vi "PH_HamamatsuCamera.set ROI Max Knob.vi"(0 "VI in":refnum<vi>, 5 "error in (no error)":errorcluster) -> (14 "VI out":refnum<vi>, 19 "error out":errorcluster)   [LabVIEW 2014, in "PH_HamamatsuCamera.lvlib"]
doc: "This VI sets several things related to ROI stuff."
uses:
  PH_HamamatsuCamera.lvlib
  PH_Common/PH_Common.lvlib
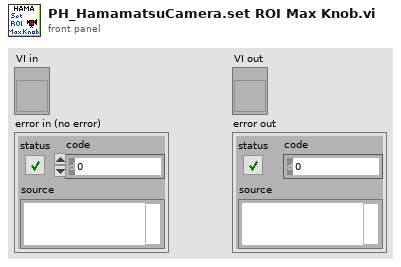
[diagram p1: front panel]
types:
  T1 = typedef "PH_HamamatsuCamera.lvlib/PH_HamamatsuCamera.i attribute.ctl" = cluster{"Gui Refs":cluster{"Camera Details":refnum<vi>, "ROI":refnum<vi>, "Set ROI to Maximum":refnum<vi>, "Trigger Parameters":refnum<vi>, "Brightness":refnum<vi>, "Shutter":refnum<vi>, "Gain":refnum<vi>, "Trigger Timeout":refnum<vi>, "Trigger Polarity":refnum<vi>, "Trigger Mode":refnum<vi>, "Parameters":refnum<vi>, "Set Cam Parameter":refnum<vi>, "Parameter to set":refnum<vi>, "Value to set":refnum<vi>}, "Cam":cluster{"Handle":i32, "Details":cluster{"Model":string, "Camera ID":string, "Firmware":string}, "Buffer Info":cluster{"height":u32, "width":u32, "datatype":u32}}, "H Offset":cluster{"Value":i32, "Minimum":i32, "Maximum":i32, "Increment":i32}, "V Offset":cluster{"Value":i32, "Minimum":i32, "Maximum":i32, "Increment":i32}, "H Width":cluster{"Value":i32, "Minimum":i32, "Maximum":i32, "Increment":i32}, "V Width":cluster{"Value":i32, "Minimum":i32, "Maximum":i32, "Increment":i32}, "Trigger Parameters":T2, "Trigger Timeout":u32, "Parameters":T3[], "Indicees Cam Parameters":cluster{"Brightness":i32, "Shutter":i32, "Gain":i32}, "Wanted Values":cluster{"Trigger Settings":T2[], "ROI":T4[], "Parameter":cluster{"Name":string, "Value":dbl}[]}}
  T2 = typedef "PH_HamamatsuCamera.lvlib/PH_HamamatsuCamera.Trigger Parameter.ctl" = cluster{"Mode":u32, "Polarity":u32, "Times":u32, "Delay":dbl}
  T3 = typedef "PH_HamamatsuCamera.lvlib/PH_HamamatsuCamera.Parameter Set.ctl" = cluster{"Parameter":string, "Value":dbl, "Writable":bool, "Range":cluster{"min":dbl, "max":dbl, "step":dbl}, "Default":dbl, "Value Names":cluster{"Name":string, "Value":dbl}[], "Text Values":bool}
  T4 = typedef "PH_HamamatsuCamera.lvlib/PH_HamamatsuCamera.ROI.ctl" = cluster{"Horizontal Offset":i32, "Vertical Offset":i32, "Horizontal Width":i32, "Vertical Width":i32}
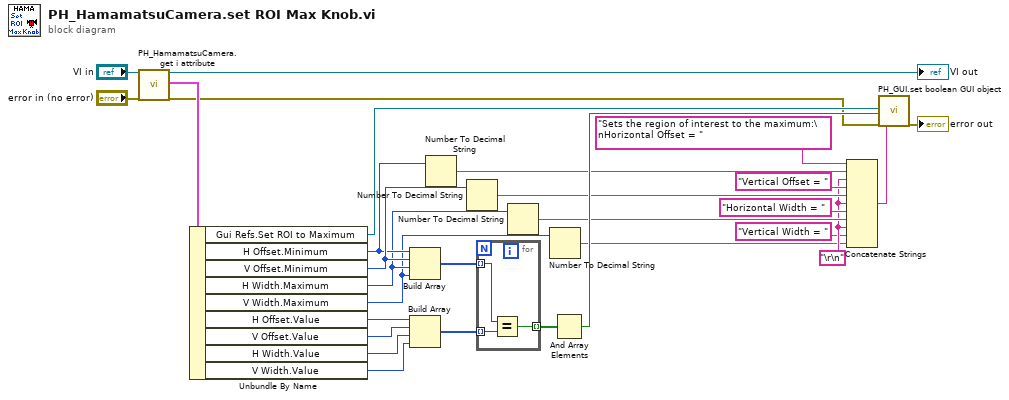
[diagram p0: block diagram]
diagram:
  w11 = "\r\n"
  n1 = call "PH_HamamatsuCamera.get i attribute.vi"("i ref in"="VI in", "error in (no error)"="error in (no error)") -> ("i ref out"=→"VI out":refnum<vi>, "i attribute"=w22:T1, "error out"=w5:errorcluster)  [unwired: 15 in]
  n2 = Unbundle By Name(w22) -> ("Gui Refs.Set ROI to Maximum"=w16:refnum<vi>, "H Offset.Minimum"=w3:i32, "V Offset.Minimum"=w4:i32, "H Width.Maximum"=w2:i32, "V Width.Maximum"=w1:i32, "H Offset.Value"=w23:i32, "V Offset.Value"=w24:i32, "H Width.Value"=w25:i32, "V Width.Value"=w26:i32)
  n3 = Build Array(w3, w4, w2, w1) -> (w17:i32[])
  n4 = Build Array(w23, w24, w25, w26) -> (w27:i32[])
  n5 = Number To Decimal String(number=w3) -> (decimal integer string=w18:string)  [unwired: 1 in]
  n6 = Number To Decimal String(number=w4) -> (decimal integer string=w14:string)  [unwired: 1 in]
  n7 = for {
    tunnel: w27 -> [w32] mode=indexing
    tunnel: w17 -> [w30] mode=indexing
    tunnel: [w31] -> w8 mode=indexing
    n8 = Equal?(x=w30, y=w32) -> (x = y?=w31:bool)
  }
  n9 = Number To Decimal String(number=w2) -> (decimal integer string=w12:string)  [unwired: 1 in]
  n10 = Number To Decimal String(number=w1) -> (decimal integer string=w9:string)  [unwired: 1 in]
  n11 = And Array Elements(Boolean array=w8) -> (logical AND=w21:bool)
  n12 = Concatenate Strings("Sets the region of interest to the maximum:\nHorizontal Offset = " ("Tip Strip"), w18, w11, "Vertical Offset = " ("string"), w14, w11, "Horizontal Width = " ("string"), w12, w11, "Vertical Width = " ("string"), w9) -> (w19:string)
  n13 = call "PH_GUI.set boolean GUI object.vi"("Boolean Knob GUI Ref"=w16, "Value"=w21, "error in (no error)"=w5, "Tip Strip"=w19) -> ("error out"=→"error out":errorcluster)  [unwired: 15 in]
